vi "Subpanel UI.vi"(8 "error in (no error)":errorcluster, 10 "Message Queue":refnum<queue>, 11 "Passive Hardware in":refnum<class "Passive Hardware.lvclass">) -> (0 "error out":errorcluster, 3 "Passive Hardware out":refnum<class "Passive Hardware.lvclass">)   [LabVIEW 2020, in "RxnRover.lvlib" / "Passive Hardware.lvclass"]
doc: "Dynamic dispatch VI that must be overridden by all inheriting classes. It is the UI that will be inserted into subpanels so data can be displayed to the user. The class will use an internally managed message queue to communicate to it. The user should only communicate to this UI through class methods."
uses:
  Passive Hardware.lvclass
  Sub VIs/Message Queue/Message Cluster.ctl
  Sub VIs/Message Queue/Enqueue Message (Single).vi
  <vilib>/Utility/error.llb/Error Cluster From Error Code.vi
  <vilib>/ErrorRing/Error Ring.xnode
  Sub VIs/Message Queue/test Message Queue.lvlib
panel:
  in  "Time Interval (sec)":i32=1200
  out "Value Graph":cluster{timestamp[], dbl[]}[](graph)
  out "Current Datapoint":dbl format="%.3f"
  out "Name":string
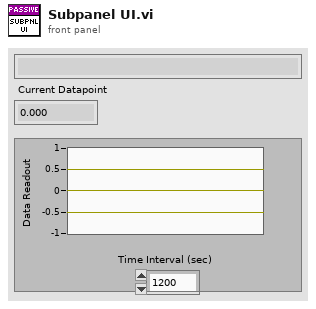
[diagram p1: front panel]
types:
  T1 = cluster{"Data Timestamps":timestamp[], "Data Values":dbl[], "Previous Run State":bool}
  T2 = typedef "RxnRover.lvlib/Passive Hardware.lvclass/Hardware State.ctl" = cluster{"VISA Resource":refnum<visa-resource-name>, "Running Since":timestamp, "Running":bool, "Sampling Rate (sec/sample)":dbl, "Data Point":cluster{"Time Stamp":timestamp, "Value":dbl}}
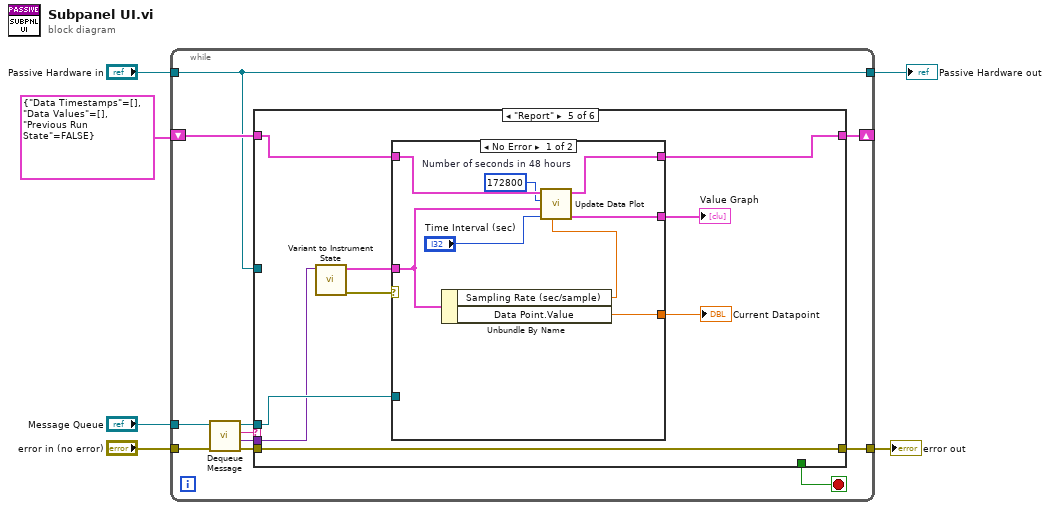
[diagram p0: block diagram]
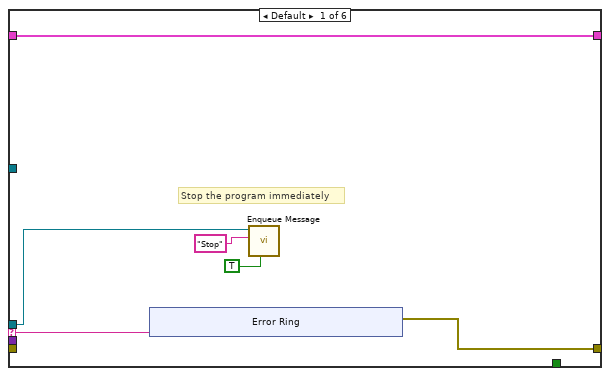
[diagram p2: hidden frame]
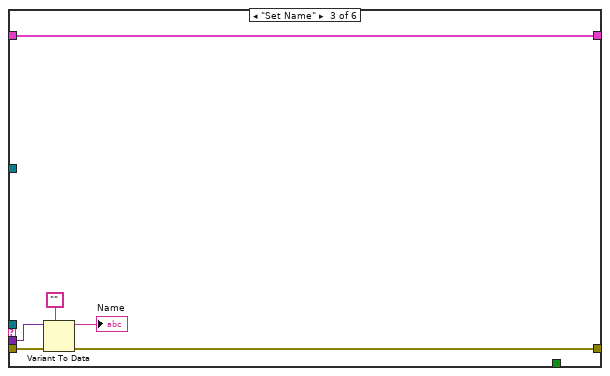
[diagram p4: hidden frame]
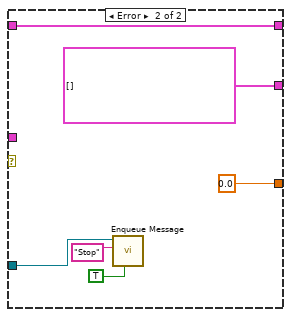
[diagram p6: hidden frame]
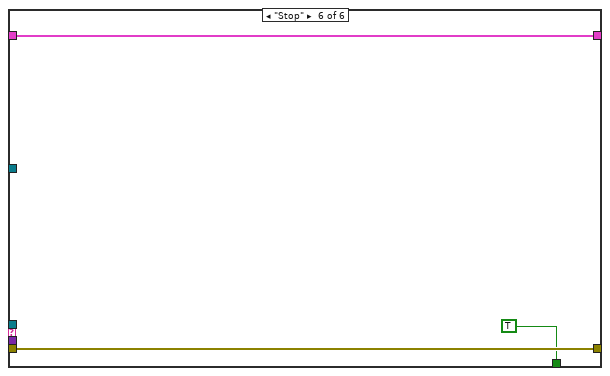
[diagram p7: hidden frame]
diagram:
  n1 = while {
    tunnel: [w7] -> w2
    tunnel: "Passive Hardware in" -> [w7]
    tunnel: [w11] -> w1
    tunnel: "error in (no error)" -> [w17]
    tunnel: "Message Queue" -> [w16]
    shift-right: [w8] -> _
    shift-left: T1 {"Data Timestamps"=[], "Data Values"=[], "Previous Run State"=FALSE} ("Graph History Arrays out") -> [w9]
    stop <- w10 stop-if-true
    n2 = call "Dequeue Message.vi"("error in (no error)"=w17, "Message Queue"=w16) -> ("error out"=w12:errorcluster, "Message Data"=w14:variant, "Message"=w15:string, "dup Message Queue"=w13:refnum<queue>)  [unwired: 6 in]
    n3 = case shown="\"Report\"" w15 {
      selector: w15 -> [w19 _ _ _ _ _]
      tunnel: w14 -> [_ _ w35 _ w42 _]
      tunnel: w13 -> [w20 _ _ _ w45 _]
      tunnel: w12 -> [_ w32 w38 w40 w49 w66]
      tunnel: [w18 w32 w36 w40 w49 w66] -> w11
      tunnel: [_ _ _ _ _ TRUE] -> w10
      tunnel: w9 -> [w23 w31 w37 w39 w48 w64]
      tunnel: [w23 w31 w37 w39 w47 w64] -> w8
      tunnel: w7 -> [_ _ _ _ _ _]
      frame Default {
        # "Stop the program immediately"
        n4 = xnode "Error Ring"("parameter 0"=w19) -> ("error out"=w18:errorcluster)
        n5 = call-poly "Enqueue Message.vi"("Priority Message? (F)"=TRUE, "Message"="Stop", "Message Queue"=w20) -> ()  [unwired: 7 in, 2 out]
      }
      frame "--- Copy this frame ---" {
      }
      frame "Set Name" {
        n6 = Variant To Data(error in=w38, type="", Variant=w35) -> (data=→"Name":string, error out=w36:errorcluster)
      }
      frame "Initialize" {
      }
      frame "Report" {
        n7 = call "Variant to Instrument State.vi"("Message Data"=w42) -> ("error out"=w46:errorcluster, "Instrument State"=w41:T2)  [unwired: 9 in]
        n8 = case shown="No Error" w46 {
          tunnel: w48 -> [w52 w63]
          tunnel: [w57 w63] -> w47
          tunnel: [w56 cluster{timestamp[], dbl[]}[] [] ("Updated Plot History")] -> w44
          tunnel: w41 -> [w55 _]
          tunnel: [w54 0.0 ("Setpoint")] -> w43
          tunnel: w45 -> [_ w60]
          frame No Error {
            w51 = 172800  # Number of seconds in 48 hours
            n9 = Unbundle By Name(w55) -> ("Sampling Rate (sec/sample)"=w50:dbl, "Data Point.Value"=w54:dbl)
            n10 = call "Update Data Plot.vi"("Sample Rate (sec/sample)"=w50, "Time interval (s)"="Time Interval (sec)", "Passive Hardware State"=w55, "History length (-1; unlimited)"=w51, "Graph History Arrays in"=w52) -> ("Updated Plot History"=w56:cluster{timestamp[], dbl[]}[], "Graph History Arrays out"=w57:T1)  [unwired: 5 in]
          }
          frame Error {
            n11 = call-poly "Enqueue Message.vi"("Priority Message? (F)"=TRUE, "Message"="Stop", "Message Queue"=w60) -> ()  [unwired: 7 in, 2 out]
          }
        }
        "Value Graph" <- w44
        "Current Datapoint" <- w43
      }
      frame "Stop" {
      }
    }
  }
  "error out" <- w1
  "Passive Hardware out" <- w2
